vi "Read Local Resource.vi"(8 "error in (no error)":errorcluster, 11 "6700C in":refnum<class "6700C.lvclass">) -> (0 "error out":errorcluster, 2 "Local Resource":refnum<visa-resource-name>, 3 "6700C out":refnum<class "6700C.lvclass">)   [LabVIEW 2019, in "6700C.lvlib" / "6700C.lvclass"]
uses:
  Library/6700C.lvclass
  Library/6700C.lvclass/6700C.ctl
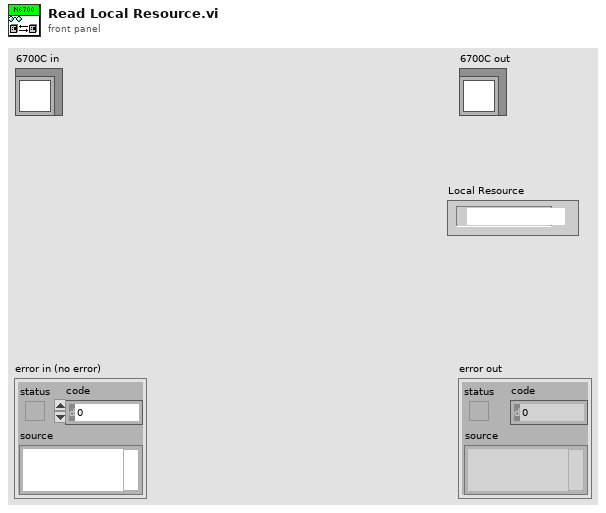
[diagram p1: front panel]
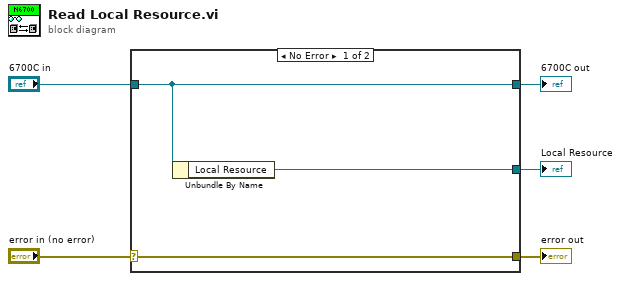
[diagram p0: block diagram]
diagram:
  n1 = case shown="No Error" "error in (no error)" {
    selector: "error in (no error)" -> [w8 w9]
    tunnel: [w8 w9] -> w4
    tunnel: [w7 w10] -> w2
    tunnel: "6700C in" -> [w7 w10]
    tunnel: [w6 _] -> w1
    frame No Error {
      n2 = Unbundle By Name(w7) -> ("Local Resource"=w6:refnum<visa-resource-name>)
    }
    frame Error {
    }
  }
  "error out" <- w4
  "6700C out" <- w2
  "Local Resource" <- w1
